vi "flip_tunnel.vi"() -> ()   [LabVIEW 2012]
uses:
  <vilib>/userdefined/High Color/IMAQdx.ctl
  <vilib>/vision/driver/IMAQdx.llb/IMAQdx Acquisition Mode.ctl
  <vilib>/Platform/TimedLoop/XDataNode/timing_clust.ctl
  <vilib>/Platform/TimedLoop/XDataNode/nitl_modes.ctl
  <vilib>/Platform/TimedLoop/XDataNode/wakeup.ctl
  <vilib>/vision/driver/IMAQdx.llb/IMAQdx Buffer Number Mode.ctl
  <vilib>/DAQmx/read.llb/DAQmx Read (Counter 1D DBL 1Chan NSamp).vi
  <vilib>/DAQmx/read.llb/DAQmx Read (Analog 1D Wfm NChan NSamp).vi
  <vilib>/DAQmx/create/channels.llb/DAQmx Create Channel (CI-Position-Angular Encoder).vi
  <vilib>/DAQmx/configure/timing.llb/DAQmx Timing (Sample Clock).vi
  <vilib>/DAQmx/create/channels.llb/DAQmx Create Channel (AI-Voltage-Basic).vi
  <vilib>/DAQmx/miscellaneous.llb/DAQmx Fill In Error Info.vi
  <vilib>/Utility/config.llb/Write Key (U32).vi
  <vilib>/Utility/config.llb/Write Key (Double).vi
  <vilib>/Utility/config.llb/Write Key (I32).vi
  <vilib>/Utility/config.llb/Write Key (String).vi
  <vilib>/platform/TimedLoop/XDataNode/XDataNode.xnode
  <resource>/objmgr/daqmx.rc
  <vilib>/vision/driver/NI_Vision_Acquisition_Software.lvlib
  <vilib>/Utility/config.llb/NI_LVConfig.lvlib
  <resource>/objmgr/imaqdx.rc
  <vilib>/Platform/TimedLoop/XDataNode/XDNodeRunTimeDep.lvlib
  <vilib>/vision/NI_Vision_Development_Module.lvlib
  <resource>/objmgr/IMAQImage.rc
panel:
  out "Speed (tunnel)":dbl(graph)
  out "Numeric":i32=1056
  out "Numeric 2":i32=1057
  out "Image CAM0- front view 3":T1(plugin-control)
  out "Lick":dbl[](graph)=[0.2311358645899357, 0.23014957542213182, 0.2311358645899357, 0.2308071015339834, 0.23047833847804877, 0.2308071015339834, 0.2311358645899357, 0.2311358645899357, 0.2308071015339834, 0.2308071015339834, 0.2308071015339834, 0.23047833847804877, 0.23014957542213182, 0.23047833847804877, 0.23047833847804877, 0.2308071015339834, 0.2308071015339834, 0.23014957542213182, 0.23047833847804877, 0.23047833847804877, 0.23047833847804877, 0.23014957542213182, 0.2298208123662325, 0.2298208123662325, 0.23047833847804877, 0.2298208123662325, 0.2298208123662325, 0.2298208123662325, 0.2298208123662325, 0.2291632862544866, 0.22949204931035078, 0.22949204931035078, 0.23014957542213182, 0.2298208123662325, 0.23014957542213182, 0.2298208123662325, 0.2298208123662325, 0.2298208123662325, 0.2298208123662325, 0.2298208123662325, 0.2298208123662325, 0.23014957542213182, 0.23014957542213182, 0.23014957542213182, 0.2298208123662325, 0.2298208123662325, 0.23047833847804877, 0.23047833847804877, 0.2298208123662325, 0.23047833847804877, 0.23014957542213182, 0.23014957542213182, 0.23014957542213182, 0.23014957542213182, 0.23014957542213182, 0.23047833847804877, 0.23014957542213182, 0.23047833847804877, 0.2308071015339834, 0.23047833847804877, 0.2298208123662325, 0.23047833847804877, 0.23047833847804877, 0.2308071015339834, 0.2308071015339834, 0.2308071015339834, 0.2311358645899357, 0.2311358645899357, 0.2311358645899357, 0.2308071015339834, 0.23047833847804877, 0.2311358645899357, 0.2311358645899357, 0.2308071015339834, 0.2308071015339834, 0.23179339070189353, 0.2308071015339834, 0.2311358645899357, 0.23146462764590575, 0.2311358645899357, 0.23146462764590575, 0.2311358645899357, 0.2311358645899357, 0.23146462764590575, 0.2311358645899357, 0.23146462764590575, 0.23146462764590575, 0.23146462764590575, 0.2311358645899357, 0.2311358645899357, 0.2311358645899357, 0.2311358645899357, 0.2311358645899357, 0.23146462764590575, 0.2308071015339834, 0.2308071015339834, 0.2308071015339834, 0.2308071015339834, 0.2308071015339834, 0.2311358645899357]
  in  "Optional Rectangle":i32[](array[numeric])=[200, 100, 550, 400]
  out "Image CAM0- front view 2":T1(plugin-control)
  out "Speed":dbl(graph)
  out "Image Type 2":i32(ring) items=["8 bits", "16 bits", "Float", "Complex", "RGB", "HSL"]
  out "Image Type":i32(ring) items=["8 bits", "16 bits", "Float", "Complex", "RGB", "HSL"]
  out "Image Size":cluster{"x":i32, "y":i32}={"x"=350, "y"=300}
  out "AISaveLoop 2":i32
  out "LEDDriver":dbl[](graph)=[-0.0036009546902470956, -0.0022859024861033913, -0.0016283763840546168, -0.0022859024861033913, -0.0026146655371335026, -0.0039297177412928146, -0.0039297177412928146, -0.00294342858816747, -0.00294342858816747, -0.0019571394350771064, -0.004587243843396215, -0.0052447699455157705, -0.00294342858816747, -0.0032721916392053243, -0.0039297177412928146, -0.0032721916392053243, -0.00294342858816747, -0.0022859024861033913, -0.0032721916392053243, -0.0032721916392053243, -0.0039297177412928146, -0.0039297177412928146, -0.00425848079234251, -0.0039297177412928146, -0.0036009546902470956, -0.0032721916392053243, -0.00425848079234251, -0.0039297177412928146, -0.0039297177412928146, -0.0039297177412928146, -0.0026146655371335026, -0.0036009546902470956, -0.0032721916392053243, -0.0026146655371335026, -0.0022859024861033913, -0.0032721916392053243, -0.0012996133330358927, -0.00294342858816747, -0.0022859024861033913, -0.0019571394350771064, -0.0019571394350771064, -0.00294342858816747, -0.0019571394350771064, -0.0016283763840546168, -0.0026146655371335026, -0.0032721916392053243, -0.0022859024861033913, -0.0032721916392053243, -0.0036009546902470956, -0.0019571394350771064, -0.0026146655371335026, -0.0039297177412928146, -0.00294342858816747, -0.00425848079234251, -0.0022859024861033913, -0.0022859024861033913, -0.0022859024861033913, -0.0026146655371335026, -0.0036009546902470956, -0.0026146655371335026, -0.0026146655371335026, -0.0026146655371335026, -0.0026146655371335026, -0.0026146655371335026, -0.00294342858816747, -0.0039297177412928146, -0.0039297177412928146, -0.00294342858816747, -0.00294342858816747, -0.00294342858816747, -0.0019571394350771064, -0.00294342858816747, -0.0019571394350771064, -0.0022859024861033913, -0.0019571394350771064, -0.0016283763840546168, -0.0036009546902470956, -0.0032721916392053243, -0.0022859024861033913, -0.0019571394350771064, -0.0009708502820209035, -0.0032721916392053243, -0.0026146655371335026, -0.00294342858816747, -0.0032721916392053243, -0.0022859024861033913, -0.0032721916392053243, -0.0026146655371335026, -0.0032721916392053243, -0.0022859024861033913, -0.0026146655371335026, -0.0026146655371335026, -0.0036009546902470956, -0.0039297177412928146, -0.0032721916392053243, -0.0026146655371335026, -0.0022859024861033913, -0.00294342858816747, -0.00294342858816747, -0.0032721916392053243]
  out "Position":dbl[](graph)=[-0.10288739642478602, -0.10288739642478602, -0.10288739642478602, -0.10288739642478602, -0.10255863337117274, -0.10255863337117274, -0.10255863337117274, -0.10288739642478602, -0.10255863337117274, -0.10288739642478602, -0.10288739642478602, -0.10321615947841241, -0.10288739642478602, -0.10288739642478602, -0.10354492253205194, -0.10321615947841241, -0.10255863337117274, -0.10321615947841241, -0.10321615947841241, -0.10354492253205194, -0.10321615947841241, -0.10387368558570464, -0.10354492253205194, -0.10387368558570464, -0.10354492253205194, -0.10321615947841241, -0.10321615947841241, -0.10354492253205194, -0.10354492253205194, -0.10354492253205194, -0.10288739642478602, -0.10420244863937056, -0.10354492253205194, -0.10321615947841241, -0.10387368558570464, -0.10321615947841241, -0.10354492253205194, -0.10354492253205194, -0.10321615947841241, -0.10321615947841241, -0.10321615947841241, -0.10321615947841241, -0.10321615947841241, -0.10288739642478602, -0.10321615947841241, -0.10387368558570464, -0.10321615947841241, -0.10321615947841241, -0.10321615947841241, -0.10321615947841241, -0.10288739642478602, -0.10321615947841241, -0.10387368558570464, -0.10321615947841241, -0.10354492253205194, -0.10354492253205194, -0.10354492253205194, -0.10354492253205194, -0.10354492253205194, -0.10321615947841241, -0.10288739642478602, -0.10321615947841241, -0.10321615947841241, -0.10288739642478602, -0.10288739642478602, -0.10255863337117274, -0.10321615947841241, -0.10288739642478602, -0.10321615947841241, -0.10321615947841241, -0.10288739642478602, -0.10255863337117274, -0.10255863337117274, -0.10288739642478602, -0.10288739642478602, -0.10354492253205194, -0.10288739642478602, -0.10321615947841241, -0.10288739642478602, -0.10288739642478602, -0.10255863337117274, -0.10255863337117274, -0.10255863337117274, -0.10255863337117274, -0.10255863337117274, -0.10288739642478602, -0.10222987031757254, -0.10222987031757254, -0.10255863337117274, -0.10288739642478602, -0.10288739642478602, -0.10255863337117274, -0.10255863337117274, -0.10255863337117274, -0.10255863337117274, -0.10255863337117274, -0.10288739642478602, -0.10288739642478602, -0.10288739642478602, -0.10288739642478602]
  out "Punish":dbl[](graph)=[-0.13181854519755057, -0.13181854519755057, -0.13214730825244975, -0.1314897821426672, -0.13214730825244975, -0.13214730825244975, -0.13247607130736472, -0.13181854519755057, -0.13247607130736472, -0.13214730825244975, -0.13181854519755057, -0.13214730825244975, -0.13214730825244975, -0.13247607130736472, -0.13214730825244975, -0.13214730825244975, -0.13247607130736472, -0.13280483436229554, -0.13280483436229554, -0.13247607130736472, -0.13247607130736472, -0.13214730825244975, -0.13247607130736472, -0.13247607130736472, -0.13247607130736472, -0.13280483436229554, -0.13247607130736472, -0.13247607130736472, -0.13280483436229554, -0.13280483436229554, -0.13247607130736472, -0.13247607130736472, -0.13247607130736472, -0.13247607130736472, -0.13313359741724223, -0.13214730825244975, -0.13247607130736472, -0.13247607130736472, -0.13247607130736472, -0.13280483436229554, -0.13280483436229554, -0.13247607130736472, -0.13280483436229554, -0.13214730825244975, -0.13280483436229554, -0.13247607130736472, -0.13247607130736472, -0.13247607130736472, -0.13280483436229554, -0.13247607130736472, -0.13247607130736472, -0.13214730825244975, -0.13247607130736472, -0.13280483436229554, -0.13247607130736472, -0.13247607130736472, -0.13247607130736472, -0.13181854519755057, -0.13247607130736472, -0.13214730825244975, -0.13247607130736472, -0.13214730825244975, -0.13247607130736472, -0.13181854519755057, -0.13247607130736472, -0.13214730825244975, -0.13214730825244975, -0.13181854519755057, -0.13214730825244975, -0.13214730825244975, -0.13214730825244975, -0.13181854519755057, -0.13181854519755057, -0.13214730825244975, -0.13181854519755057, -0.13214730825244975, -0.1311610190877996, -0.1314897821426672, -0.1314897821426672, -0.13181854519755057, -0.1314897821426672, -0.13181854519755057, -0.13214730825244975, -0.1314897821426672, -0.1314897821426672, -0.1314897821426672, -0.13214730825244975, -0.13181854519755057, -0.13214730825244975, -0.13181854519755057, -0.13214730825244975, -0.13181854519755057, -0.13214730825244975, -0.13181854519755057, -0.13247607130736472, -0.1314897821426672, -0.13214730825244975, -0.13181854519755057, -0.13181854519755057, -0.13181854519755057]
  out "FramePulse":dbl[](graph)=[-0.0019571394350771064, -0.0016283763840546168, -0.0006420872310096188, -0.0012996133330358927, -0.0006420872310096188, -0.0012996133330358927, -0.0022859024861033913, -0.0022859024861033913, -0.0022859024861033913, -0.0026146655371335026, -0.00425848079234251, -0.0032721916392053243, -0.0019571394350771064, -0.0039297177412928146, -0.00425848079234251, -0.0006420872310096188, -0.0016283763840546168, -0.0019571394350771064, -0.0036009546902470956, -0.0022859024861033913, -0.0036009546902470956, -0.0022859024861033913, -0.0032721916392053243, -0.0022859024861033913, -0.0032721916392053243, -0.00294342858816747, -0.0036009546902470956, -0.0022859024861033913, -0.0016283763840546168, -0.0026146655371335026, -0.0016283763840546168, -0.0026146655371335026, -0.00294342858816747, -0.0006420872310096188, -0.0019571394350771064, -0.00294342858816747, -0.0009708502820209035, -0.0022859024861033913, -0.0009708502820209035, -0.0019571394350771064, -0.0012996133330358927, -0.0039297177412928146, -0.0026146655371335026, -0.0012996133330358927, -0.0012996133330358927, -0.0019571394350771064, -0.00294342858816747, -0.0022859024861033913, -0.00294342858816747, -0.0026146655371335026, -0.0019571394350771064, -0.0019571394350771064, -0.00294342858816747, -0.0036009546902470956, -0.0012996133330358927, -0.00031332418000200855, -0.0016283763840546168, -0.0019571394350771064, -0.00294342858816747, -0.0026146655371335026, -0.0036009546902470956, -0.0022859024861033913, -0.0019571394350771064, -0.0006420872310096188, -0.0009708502820209035, -0.0026146655371335026, -0.0036009546902470956, -0.0009708502820209035, -0.0026146655371335026, -0.0032721916392053243, -0.0019571394350771064, -0.00294342858816747, -0.0019571394350771064, -0.0022859024861033913, -0.00294342858816747, -0.0022859024861033913, -0.0036009546902470956, -0.0016283763840546168, -0.0026146655371335026, -0.0016283763840546168, -0.0019571394350771064, -0.0022859024861033913, -0.0019571394350771064, -0.0016283763840546168, -0.0022859024861033913, -0.0012996133330358927, -0.0012996133330358927, -0.0016283763840546168, -0.0012996133330358927, -0.0022859024861033913, -0.0026146655371335026, -0.0016283763840546168, -0.0032721916392053243, -0.0036009546902470956, -0.0019571394350771064, -0.0012996133330358927, -0.0016283763840546168, -0.0012996133330358927, -0.0019571394350771064, -0.0019571394350771064]
  out "Stim ID":dbl[](graph)=[-0.2067765221829541, -0.2067765221829541, -0.2067765221829541, -0.2067765221829541, -0.2064477591236867, -0.20710528524224417, -0.2067765221829541, -0.2067765221829541, -0.20710528524224417, -0.20710528524224417, -0.20710528524224417, -0.2067765221829541, -0.2067765221829541, -0.20710528524224417, -0.2067765221829541, -0.20710528524224417, -0.20710528524224417, -0.20710528524224417, -0.20743404830155698, -0.2067765221829541, -0.20710528524224417, -0.20710528524224417, -0.20710528524224417, -0.2067765221829541, -0.20743404830155698, -0.2067765221829541, -0.20710528524224417, -0.2064477591236867, -0.20710528524224417, -0.2067765221829541, -0.2067765221829541, -0.20710528524224417, -0.2067765221829541, -0.2064477591236867, -0.2067765221829541, -0.20710528524224417, -0.20710528524224417, -0.20743404830155698, -0.20710528524224417, -0.2067765221829541, -0.2067765221829541, -0.20710528524224417, -0.2067765221829541, -0.2067765221829541, -0.2067765221829541, -0.20710528524224417, -0.2067765221829541, -0.2067765221829541, -0.2064477591236867, -0.20743404830155698, -0.2067765221829541, -0.20710528524224417, -0.2067765221829541, -0.2067765221829541, -0.20710528524224417, -0.20710528524224417, -0.20743404830155698, -0.20743404830155698, -0.20710528524224417, -0.20710528524224417, -0.2067765221829541, -0.20710528524224417, -0.20710528524224417, -0.2067765221829541, -0.2064477591236867, -0.20710528524224417, -0.2067765221829541, -0.20743404830155698, -0.2067765221829541, -0.2064477591236867, -0.2064477591236867, -0.2067765221829541, -0.2064477591236867, -0.2067765221829541, -0.20710528524224417, -0.2064477591236867, -0.20710528524224417, -0.2067765221829541, -0.2067765221829541, -0.2067765221829541, -0.2067765221829541, -0.2067765221829541, -0.20710528524224417, -0.2067765221829541, -0.2067765221829541, -0.2067765221829541, -0.2067765221829541, -0.2067765221829541, -0.2064477591236867, -0.2067765221829541, -0.20743404830155698, -0.2064477591236867, -0.2067765221829541, -0.2064477591236867, -0.20743404830155698, -0.20710528524224417, -0.20710528524224417, -0.2064477591236867, -0.20743404830155698, -0.2067765221829541]
  out "Photodiode":dbl[](graph)=[1.0477834277971203, 1.0444957958656487, 1.0550162180791747, 1.0579750868439877, 1.0694817987797698, 1.0790159316147676, 1.088878827735934, 1.0796734580201486, 1.0970979079034913, 1.099728013569978, 1.098741723944312, 1.0842761428685865, 1.0895363541471035, 1.0800022212229832, 1.0497560069604706, 1.0283863995350169, 1.048769717378376, 1.0435095062880182, 1.0481121909907791, 1.0494272437663457, 1.0329890841783826, 1.0517285861271792, 1.0395643479858325, 1.0602764292218856, 1.0369342424584334, 1.0803309844259137, 1.0803309844259137, 1.0892075909414702, 1.088878827735934, 1.099728013569978, 1.0957828550725925, 1.0895363541471035, 1.0763858259970813, 1.0760570627953017, 1.073426957184508, 1.0550162180791747, 1.0339753737471549, 1.0435095062880182, 1.0408794007517477, 1.0438382694804689, 1.0227974253492698, 1.0467971382167025, 1.0553449812748896, 1.0648791139915486, 1.0494272437663457, 1.0760570627953017, 1.0878925381199063, 1.0908514069706063, 1.0898651173528338, 1.0517285861271792, 1.0924952230021696, 1.0901938805586608, 1.0829610900528213, 1.064550350793101, 1.0599476660247606, 1.0586326132372021, 1.0553449812748896, 1.0402218743686054, 1.0339753737471549, 1.0405506375601303, 1.0438382694804689, 1.038578058412366, 1.0513998229324943, 1.0513998229324943, 1.0655366403887276, 1.0711256147800765, 1.0790159316147676, 1.0875637749147575, 1.0763858259970813, 1.100056776778729, 1.0872350117097054, 1.0859199588904642, 1.0842761428685865, 1.0744132467878387, 1.052714875711795, 1.0507422965434046, 1.0507422965434046, 1.045810848637122, 1.0303589786656915, 1.0362767160775053, 1.0379205320305165, 1.0264138204076296, 1.0441670326730124, 1.0612627188138266, 1.064221587594748, 1.0727694307827649, 1.0704680883796682, 1.0892075909414702, 1.0892075909414702, 1.081974800442009, 1.073426957184508, 1.0892075909414702, 1.081974800442009, 1.0707968515798247, 1.0237837149095494, 1.0467971382167025, 1.0513998229324943, 1.0313452682322635, 1.03759176883973, 1.0178659775601138]
  out "Elapsed time":u32=37 format="%<%H:%M:%S>t"
  in  "?":enum32{"CodePerformance", "SetPath"}(tab)=enum."SetPath"
  out "CamerasOK? TaskEnd OK?":errorcluster
  in  "SetPath OK?":errorcluster
  out "AcqLoopRes[ms]":u32=100
  out "SaveLoopRes[ms]":u32=100
  out "AISaveLoop":i32=373
  out "AIAcqLoop":i32=372
  out "Cam2AcqRes[ms]":u32=40
  out "# elements in queue":i32
  out "Cam1AcqRes[ms]":u32=63
  out "error out":errorcluster
  out "Buffer Number  2":u32=1189
  out "Frame Rate 2":dbl=28.403525954946133
  out "Buffer Number":u32=47166
  out "Frame Rate":dbl=15.968063872255488
  in  "File prefix":string="T7"
  in  "Path":path=path "D:/Kelly_Raja"
  out "FileName":string="20170427_193446_T7"
  out "byte order (0:big-endian, network order)":T2(ring)
  out "NumChans":u32=12
  in  "SaveData":bool
  in  "all stop":bool=TRUE
  in  "start":bool=TRUE
  in  "samples per channel":i32=100
  in  "rate":dbl=1000.0 format="%0.2f"
  out "Acquired Frames CAM0":dbl=28.431372549019606
  out "SaveLoopRes[ms] 2":u32=348059
  out "# elements in queue 2":i32
  out "Number of trials":dbl
  out "?":T1(plugin-control)
  out "?":T1(plugin-control)
  out "Reward":dbl[](graph)=[1.543887100195785e-05, -0.00031332418000200855, 1.543887100195785e-05, 1.543887100195785e-05, -0.00031332418000200855, -0.00031332418000200855, 0.0003442019220023107, 1.543887100195785e-05, 0.0003442019220023107, 0.0003442019220023107, 1.543887100195785e-05, 0.0003442019220023107, 1.543887100195785e-05, 1.543887100195785e-05, 1.543887100195785e-05, -0.00031332418000200855, -0.00031332418000200855, 1.543887100195785e-05, -0.00031332418000200855, 0.0003442019220023107, -0.0006420872310096188, 1.543887100195785e-05, 1.543887100195785e-05, 0.0003442019220023107, 1.543887100195785e-05, 0.0003442019220023107, 0.0003442019220023107, -0.0006420872310096188, 1.543887100195785e-05, 1.543887100195785e-05, 0.0003442019220023107, -0.00031332418000200855, 1.543887100195785e-05, 1.543887100195785e-05, 1.543887100195785e-05, 1.543887100195785e-05, 0.0003442019220023107, 1.543887100195785e-05, 1.543887100195785e-05, 0.0003442019220023107, -0.00031332418000200855, 1.543887100195785e-05, 1.543887100195785e-05, 1.543887100195785e-05, 1.543887100195785e-05, 0.0003442019220023107, -0.00031332418000200855, -0.0006420872310096188, 1.543887100195785e-05, 1.543887100195785e-05, 1.543887100195785e-05, 1.543887100195785e-05, 1.543887100195785e-05, 0.0003442019220023107, 1.543887100195785e-05, 1.543887100195785e-05, -0.00031332418000200855, -0.00031332418000200855, 1.543887100195785e-05, -0.00031332418000200855, -0.00031332418000200855, 1.543887100195785e-05, 1.543887100195785e-05, 1.543887100195785e-05, 1.543887100195785e-05, 0.0003442019220023107, 1.543887100195785e-05, -0.00031332418000200855, -0.00031332418000200855, -0.00031332418000200855, 1.543887100195785e-05, 0.0003442019220023107, 1.543887100195785e-05, -0.00031332418000200855, 1.543887100195785e-05, 1.543887100195785e-05, 0.0006729649729990802, 1.543887100195785e-05, 1.543887100195785e-05, 0.0003442019220023107, -0.00031332418000200855, -0.00031332418000200855, 1.543887100195785e-05, 0.0003442019220023107, 1.543887100195785e-05, 1.543887100195785e-05, -0.00031332418000200855, 1.543887100195785e-05, 1.543887100195785e-05, -0.00031332418000200855, 0.0003442019220023107, -0.00031332418000200855, 1.543887100195785e-05, 1.543887100195785e-05, 1.543887100195785e-05, 1.543887100195785e-05, 1.543887100195785e-05, -0.00031332418000200855, -0.00031332418000200855, -0.00031332418000200855]
  out "dup path":path=path "D:/Kelly_Raja"
  out "created path":path=path "D:/Kelly_Raja"
  # "RecordAI_VI (orsolici, 2016)"
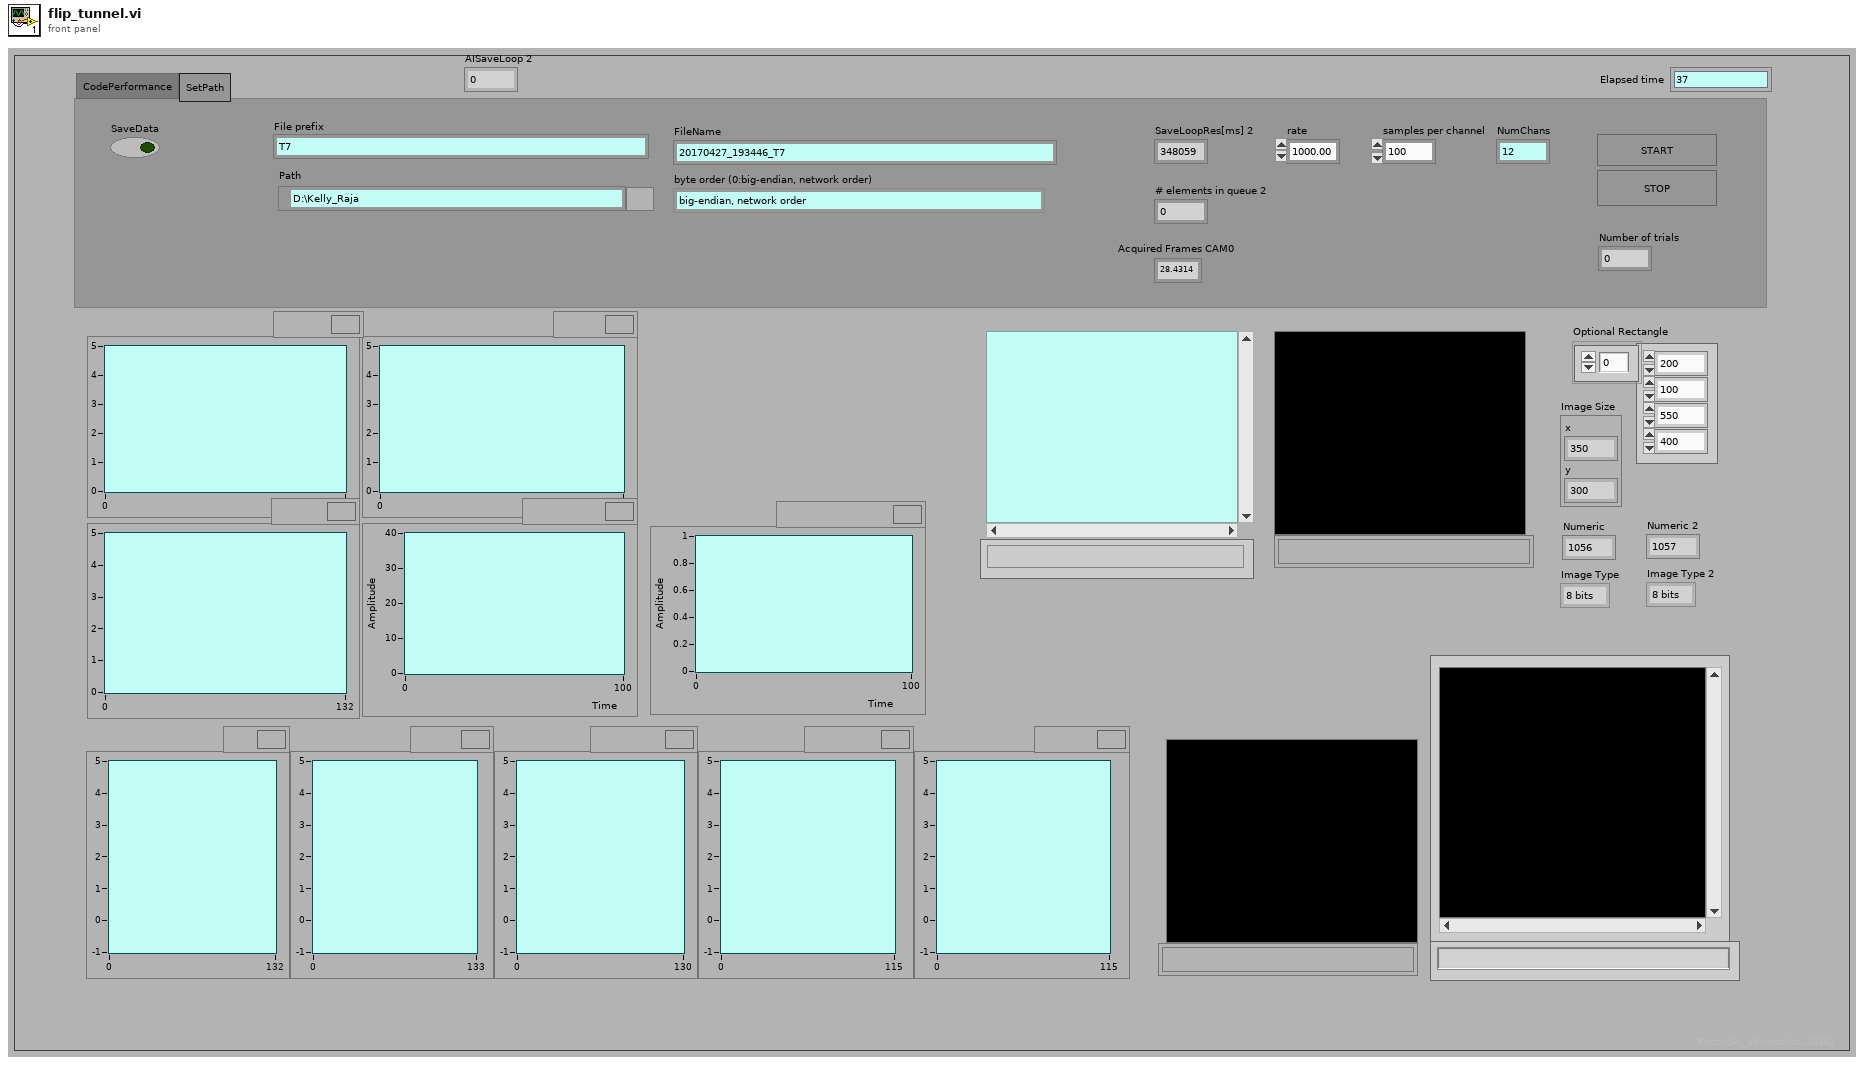
[diagram p1: front panel]
types:
  T1 = typedef "IMAQ Image.ctl" = refnum<image>
  T2 = enum16{"big-endian, network order", "native, host order", "little-endian"}
  T3 = typedef "IMAQdx.ctl" = refnum<k21>
  T4 = typedef "Image Type" = u32
  T5 = cluster{i32, "millisecond timer value":u32, "Buffer Number Out":u32, "Image Pixels (U8)":u8[][]}
  T6 = cluster{"data":waveform(dbl)[], "data":dbl[], "millisecond timer value":u32, i32}
  T7 = typedef "NI_Vision_Acquisition_Software.lvlib/IMAQdx Acquisition Mode.ctl" = enum32{"One Shot", "Continuous"}
  T8 = cluster{"New Image":T1, "Session Out":T3, "error out":errorcluster}
  T9 = cluster{"task out":refnum<k21>, "error out":errorcluster, "task out":refnum<k21>, "error out":errorcluster}
  T10 = cluster{"Session Out":T3, "New Image":T1, "New Image":T1, "error out":errorcluster}
  T11 = typedef "XDNodeRunTimeDep.lvlib/timing_clust.ctl" = cluster{"Expected End [f-1]":u64, "Actual End [f-1]":u64, "Finished Late? [f-1]":bool, "Expected End [i-1]":u64, "Actual End [i-1]":u64, "Finished Late? [i-1]":bool, "Expected Start [i]":u64, "Actual Start [i]":u64, "Expected Start [f]":u64, "Actual Start [f]":u64, "Source Name":string, "Structure Name":string, "Period":i64, "Deadline":i64, "Offset":i64, "Start":i64, "Priority":i32, "Timeout":i32, "Mode":T12, "Wakeup Reason":T13, "Error":errorcluster, "Source Type":string, "Secondary Source Type":string, "Global End Time":u64, "Global Start Time":u64, "Frame Duration":u64, "Iteration Duration":u64, "Assigned CPU":i32, "I/O Scan Engine Mode":u32}
  T12 = typedef "XDNodeRunTimeDep.lvlib/nitl_modes.ctl" = enum32{"No Change", "Process missed periods, maintain original phase", "Discard missed periods, maintain original phase", "Process missed periods, ignore original phase", "Discard missed periods, ignore original phase"}
  T13 = typedef "XDNodeRunTimeDep.lvlib/wakeup.ctl" = enum32{"Normal", "Aborted", "Asynchronous wakeup", "Timing source error", "Timed loop error", "Timeout"}
  T14 = enum16{"open", "replace", "create", "open or create", "replace or create", "replace or create with confirmation"}
  T15 = cluster{refnum<file>[], "refnum out":refnum<file>, "refnum out":refnum<file>, "refnum out":refnum<file>}
  T16 = typedef "NI_Vision_Acquisition_Software.lvlib/IMAQdx Buffer Number Mode.ctl" = enum32{"Next", "Last", "Buffer Number"}
  T17 = cluster{"Image Out":T1, "Session Out":T3, "error out":errorcluster}
  T18 = cluster{"Session Out":T3, "error out":errorcluster, "New Image":T1}
  T19 = cluster{cluster{"Image Out":T1, "Session Out":T3, "error out":errorcluster}, cluster{"Image Out":T1, "Session Out":T3, "error out":errorcluster}}
  T20 = typedef "NI_LVConfig.lvlib/Config Data RefNum.ctl" = refnum<k1>
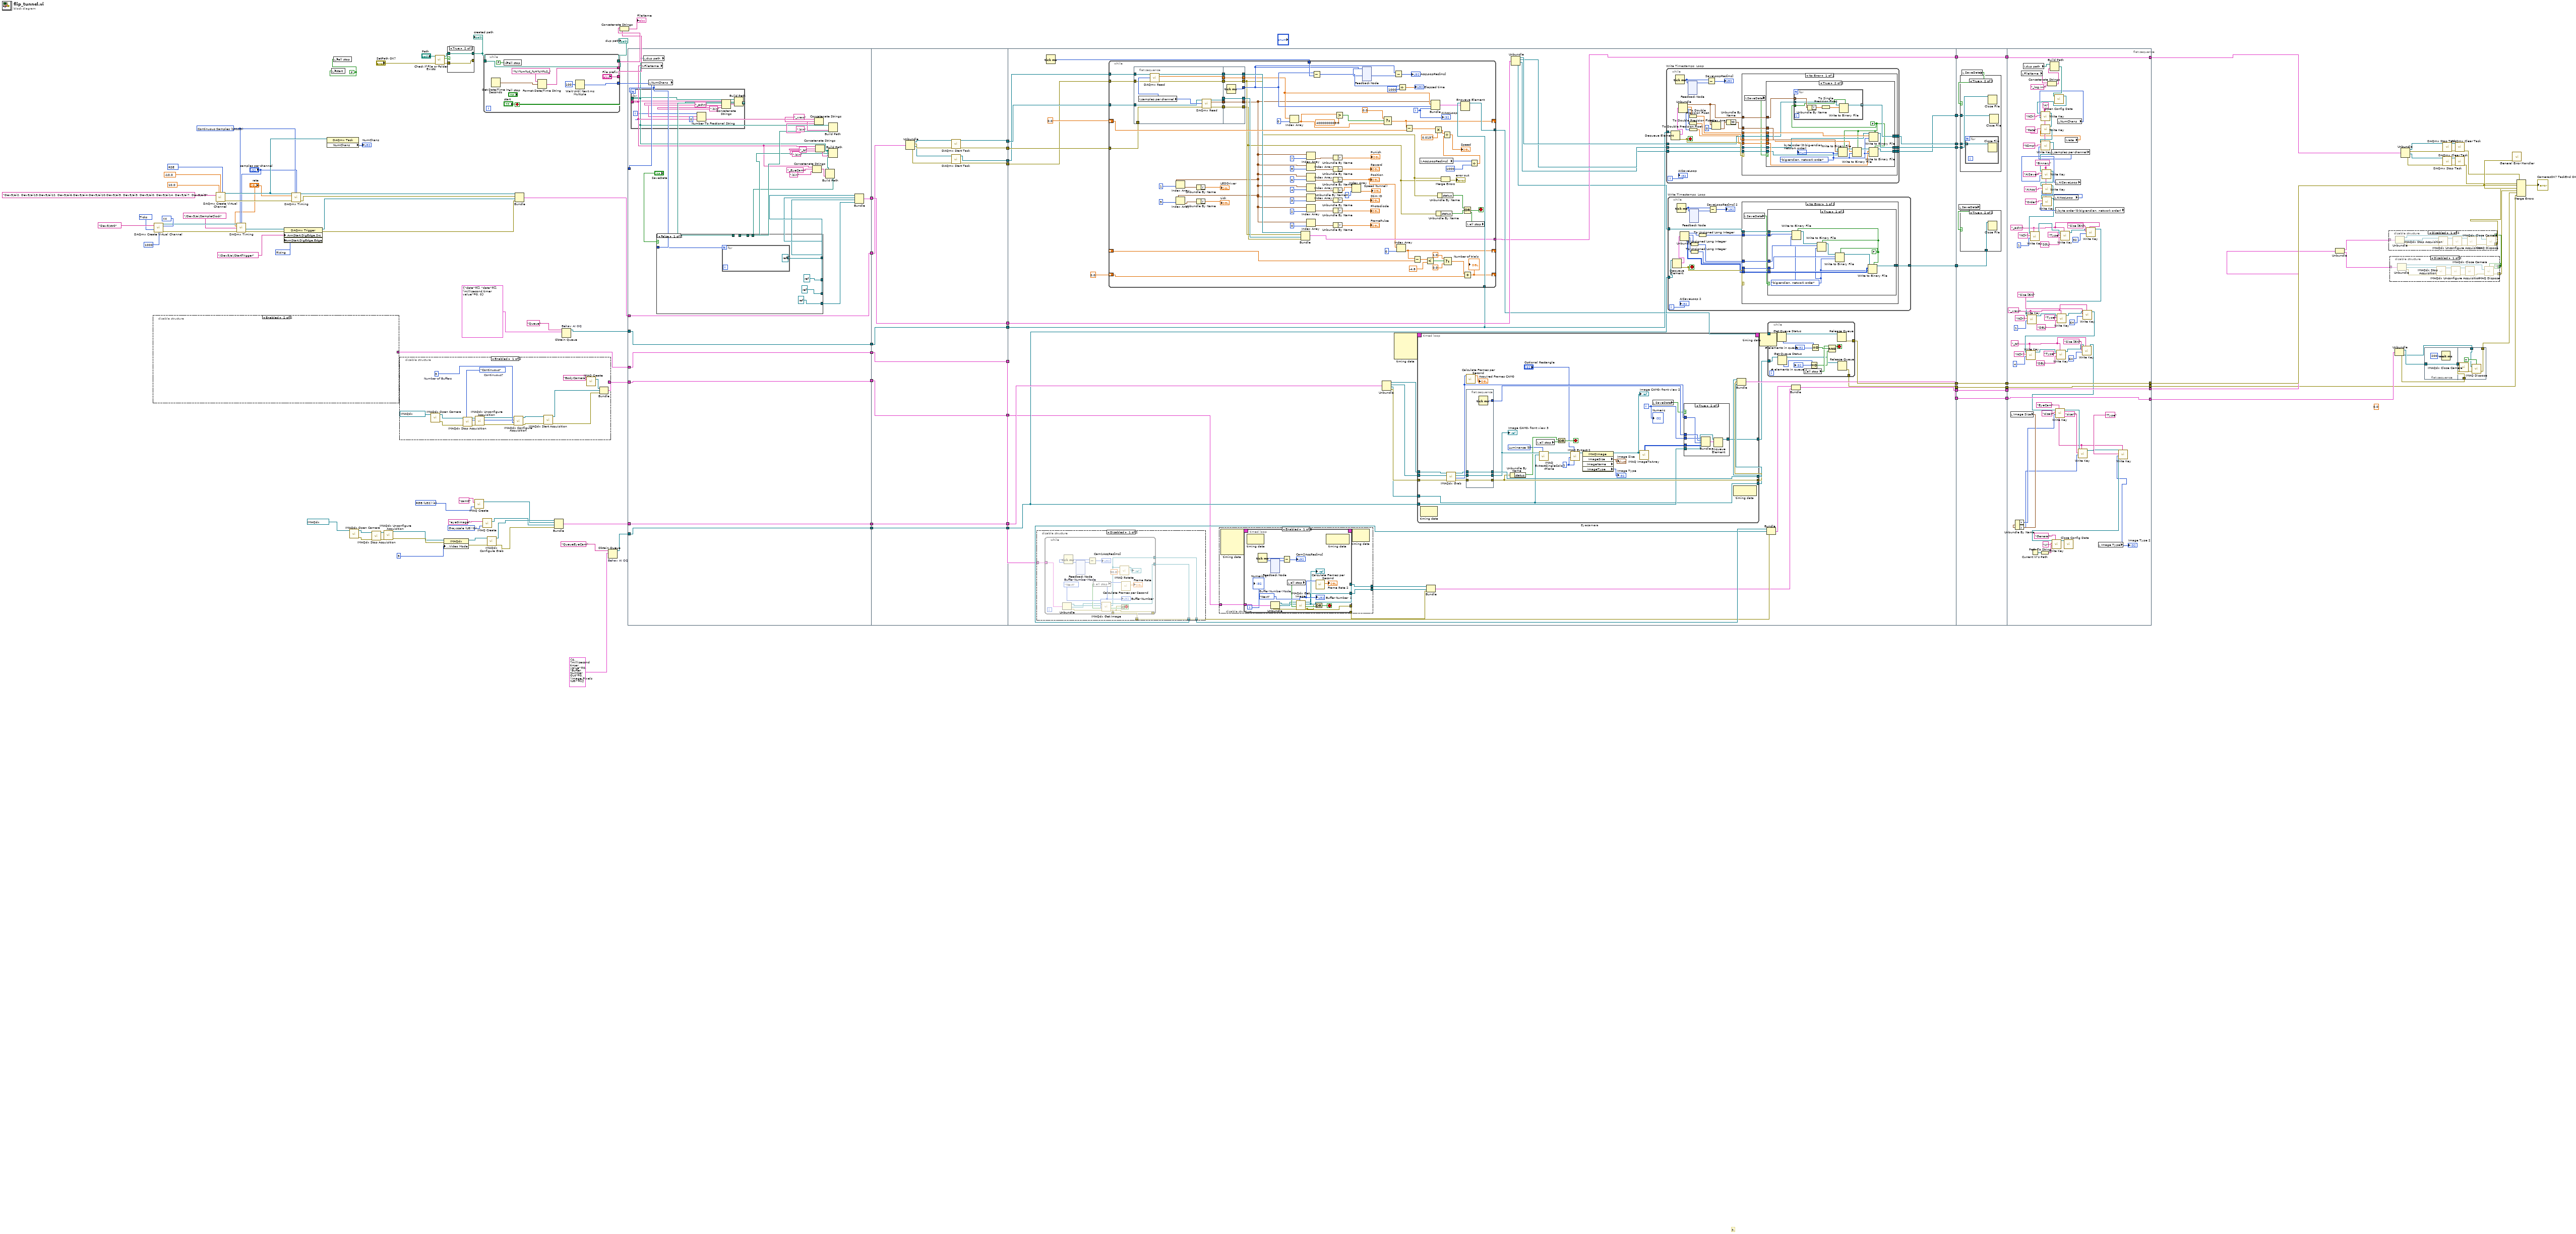
[diagram p0: block diagram]
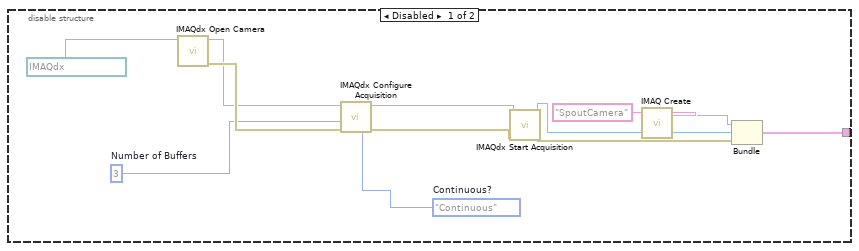
[diagram p5: hidden frame]
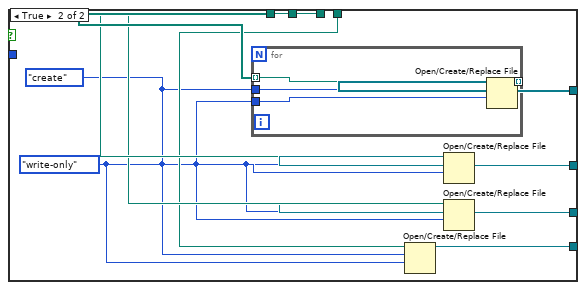
[diagram p6: hidden frame]
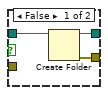
[diagram p16: hidden frame]
diagram:
  w30 = T4 0 items=["Grayscale (U8)", "Grayscale (I16)", "Grayscale (SGL)", "Complex (CSG)", "RGB (U32)", "HSL (U32)", "RGB (U64)", "Grayscale (U16)"] ("Image Type")
  w32 = T4 4 items=["Grayscale (U8)", "Grayscale (I16)", "Grayscale (SGL)", "Complex (CSG)", "RGB (U32)", "HSL (U32)", "RGB (U64)", "Grayscale (U16)"] ("Image Type")
  (unwired) 0.0 ("data")
  w59 = 10304 items=["Degrees"=10146, "Radians"=10273, "Ticks"=10304, "From Custom Scale"=10065] ("units")
  w2 = 10123 items=["Finite Samples"=10178, "Continuous Samples"=10123, "Hardware Timed Single Point"=12522] ("sample mode")
  w73 = 10083 items=["default"=-1, "RSE"=10083, "NRSE"=10078, "Differential"=10106, "Pseudodifferential"=12529] ("input terminal configuration")
  w70 = 10092 items=["X1"=10090, "X2"=10091, "X4"=10092, "Two Pulse Counting"=10313] ("E1 decoding type")
  w63 = 10280 items=["Rising"=10280, "Falling"=10171] ("ArmStart.DigEdge.Edge")
  w13 = FALSE
  # "3."
  n1 = disable-structure shown="Enabled" {
    disable-tunnel: [w130 _] -> w100
    frame Disabled {
      w123 = IMAQdx_Acquisition_Mode."Continuous"  # Continuous?
      w133 = u32 3  # Number of Buffers
      n2 = call <vilib>:"IMAQdx Open Camera.vi"("Session In"=T3 "spout camera" ("Camera1")) -> ("error out"=w134:errorcluster, "Session Out"=w129:T3)  [unwired: 2 in, 7 out]
      n3 = call <vilib>:"IMAQdx Configure Acquisition.vi"("error in"=w134, "Number of Buffers"=w133, "Continuous?"=w123, "Session In"=w129) -> ("error out"=w124:errorcluster, "Session Out"=w127:T3)  [unwired: 6 out]
      n4 = call <vilib>:"IMAQdx Start Acquisition.vi"("error in"=w124, "Session In"=w127) -> ("error out"=w125:errorcluster, "Session Out"=w126:T3)  [unwired: 8 out]
      n5 = call "IMAQ Create"("Image Name"="SpoutCamera") -> ("New Image"=w131:T1)  [unwired: 3 in, 2 out]
      n6 = Bundle("New Image"=w131, "Session Out"=w126, "error out"=w125) -> (w130:T8)  [unwired: 1 in]
    }
    frame Enabled {
    }
  }
  n7 = call-poly <vilib>:"DAQmx Create Virtual Channel.vi"("counter"=tag "Dev5/ctr0" ("E1 counter"), "decoding type"=w70, "units"=w59, "pulses per revolution"=u32 1000 ("E1 pulses per revolution")) -> ("task out"=w68:refnum<k21>, "error out"=w67:errorcluster)  [unwired: 10 in]
  n8 = call-poly <vilib>:"DAQmx Create Virtual Channel.vi"("maximum value"=10.0, "minimum value"=-10.0, "input terminal configuration"=w73, "physical channels"=tag "Dev5/ai2, Dev5/ai13,Dev5/ai12, Dev5/ai6,Dev5/ai4,Dev5/ai10,Dev5/ai5, Dev5/ai3, Dev5/ai0, Dev5/ai14, Dev5/ai7, Dev5/ai9" ("Analogue Input Channel")) -> ("task out"=w62:refnum<k21>, "error out"=w72:errorcluster)  [unwired: 10 in]
  n9 = call-poly <vilib>:"DAQmx Timing.vi"("task/channels in"=w68, "sample mode"=w2, "samples per channel"="samples per channel", "rate"="rate", "source"=tag "/Dev5/ai/SampleClock", "error in"=w67) -> ("task out"=w65:refnum<k21>, "error out"=w64:errorcluster)  [unwired: 8 in]
  n10 = property class="DAQmx Trigger"(reference=w65, error in=w64, "ArmStart.DigEdge.Src"=tag "/Dev5/ai/StartTrigger", "ArmStart.DigEdge.Edge"=w63) -> (reference out=w56:refnum<k21>, error out=w55:errorcluster)
  n11 = call-poly <vilib>:"DAQmx Timing.vi"("task/channels in"=w62, "sample mode"=w2, "samples per channel"="samples per channel", "rate"="rate", "error in"=w72) -> ("task out"=w58:refnum<k21>, "error out"=w57:errorcluster)  [unwired: 9 in]
  n12 = property class="DAQmx Task"(reference=w62) -> ("NumChans"=→"NumChans":u32)  [unwired: 1 in, 2 out]
  n13 = local write "start"(w13) -> ()
  n14 = local write "all stop"(w13) -> ()
  n15 = call <vilib>:"IMAQdx Open Camera.vi"("Session In"=T3 "eyecam2") -> ("error out"=w5:errorcluster, "Session Out"=w7:T3)  [unwired: 2 in, 7 out]
  n16 = call <vilib>:"IMAQdx Stop Acquisition.vi"("error in"=w5, "Session In"=w7) -> ("error out"=w4:errorcluster, "Session Out"=w6:T3)  [unwired: 8 in]
  n17 = call <vilib>:"IMAQdx Unconfigure Acquisition.vi"("error in"=w4, "Session In"=w6) -> ("error out"=w34:errorcluster, "Session Out"=w33:T3)  [unwired: 8 out]
  n18 = disable-structure shown="Enabled" {
    disable-tunnel: [w141 _] -> w10
    frame Enabled {
      w143 = u32 3  # Number of Buffers
      w145 = IMAQdx_Acquisition_Mode."Continuous"  # Continuous?
      n19 = call <vilib>:"IMAQdx Open Camera.vi"("Session In"=T3 "mousecam" ("Camera2")) -> ("error out"=w137:errorcluster, "Session Out"=w138:T3)  [unwired: 2 in, 7 out]
      n20 = call <vilib>:"IMAQdx Stop Acquisition.vi"("error in"=w137, "Session In"=w138) -> ("error out"=w140:errorcluster, "Session Out"=w139:T3)  [unwired: 8 in]
      n21 = call <vilib>:"IMAQdx Unconfigure Acquisition.vi"("error in"=w140, "Session In"=w139) -> ("error out"=w135:errorcluster, "Session Out"=w136:T3)  [unwired: 8 out]
      n22 = call <vilib>:"IMAQdx Configure Acquisition.vi"("error in"=w135, "Number of Buffers"=w143, "Continuous?"=w145, "Session In"=w136) -> ("error out"=w148:errorcluster, "Session Out"=w147:T3)  [unwired: 6 out]
      n23 = call <vilib>:"IMAQdx Start Acquisition.vi"("error in"=w148, "Session In"=w147) -> ("error out"=w149:errorcluster, "Session Out"=w150:T3)  [unwired: 8 out]
      n24 = call "IMAQ Create"("Image Name"="BodyCamera") -> ("New Image"=w144:T1)  [unwired: 3 in, 2 out]
      n25 = Bundle("New Image"=w144, "Session Out"=w150, "error out"=w149) -> (w141:T8)  [unwired: 1 in]
    }
    frame Disabled {
    }
  }
  n26 = call <vilib>:"Check if File or Folder Exists.vi"("error in (no error)"="SetPath OK?", "path"="Path") -> ("error out"=w118:errorcluster, "file or folder exists?"=w122:bool, "dup path"=w121:path)  [unwired: 7 in]
  n27 = property class="IMAQdx"(reference=w33, error in=w34, "Acquisition Attributes:Video Mode"=u32 5 ("VideoMode")) -> (reference out=w36:T3, error out=w35:errorcluster)
  n28 = case shown="True" w122 {
    tunnel: w121 -> [w153 w155]
    tunnel: [w152 w155] -> w119
    tunnel: w118 -> [_ w154]
    tunnel: [w151 w154] -> _
    frame False {
      n29 = Create Folder(path (use dialog)=w153) -> (created path=w152:path, error out=w151:errorcluster)  [unwired: 2 in, 1 out]
    }
    frame True {
    }
  }
  "created path" <- w119
  n30 = call "IMAQ Create"("Image Name"="cam0", "Image Type"=w32) -> ("New Image"=w41:T1)  [unwired: 2 in, 2 out]
  n31 = call "IMAQ Create"("Image Name"="eye0image", "Image Type"=w30) -> ("New Image"=w40:T1)  [unwired: 3 in, 1 out]
  n32 = while {
    tunnel: w119 -> [w156]
    tunnel: [w159] -> w102
    tunnel: ["File prefix"] -> w116
    tunnel: [w161] -> w117
    tunnel: [w156] -> w114
    stop <- "start" stop-if-true
    n33 = Get Date/Time In Seconds() -> (seconds since 1Jan1904=w157:timestamp)
    n34 = local write "all stop"(FALSE ("stop")) -> ()
    n35 = Format Date/Time String(time format string (%c)="%Y%m%d_%H%M%S_", seconds (now)=w157) -> (date/time string=w161:string)  [unwired: 1 in]
    n36 = Wait Until Next ms Multiple(millisecond multiple=u32 100) -> (millisecond timer value=w159:u32)
  }
  "dup path" <- w114
  n37 = call <vilib>:"IMAQdx Configure Grab.vi"("error in"=w35, "Session In"=w36) -> ("error out"=w53:errorcluster, "Session Out"=w42:T3)  [unwired: 1 in, 7 out]
  n38 = Bundle("task out"=w58, "error out"=w57, "task out"=w56, "error out"=w55) -> (w61:T9)  [unwired: 1 in]
  n39 = Bundle("Session Out"=w42, "New Image"=w41, "New Image"=w40, "error out"=w53) -> (w52:T10)  [unwired: 1 in]
  n40 = Obtain Queue "Behav AI OQ"(name (unnamed)="Queue", element data type=T6 {"data"=[], "data"=[], "millisecond timer value"=0, 0} ("cluster")) -> (queue out=w110:refnum<queue>)  [unwired: 3 in, 2 out]
  n41 = Obtain Queue "Behav AI OQ"(name (unnamed)="QueueEyeCam", element data type=T5 {0, "millisecond timer value"=0, "Buffer Number Out"=0, "Image Pixels (U8)"=[]} ("output cluster")) -> (queue out=w45:refnum<queue>)  [unwired: 3 in, 2 out]
  n42 = Concatenate Strings(w117, w116) -> (→"FileName":string)
  n43 = flat-sequence {
    tunnel: [w186] -> w111
    tunnel: w110 -> [w185]
    tunnel: [w185] -> w109
    tunnel: w102 -> [_]
    tunnel: w100 -> [w176]
    tunnel: [w176] -> w99
    tunnel: w61 -> [w177]
    tunnel: [w177] -> w95
    tunnel: [w165] -> w89
    tunnel: w52 -> [w174]
    tunnel: [w174] -> w50
    tunnel: w45 -> [w173]
    tunnel: [w173] -> w44
    tunnel: w10 -> [w165]
    tunnel: [w236] -> w112
    tunnel: w111 -> [w236]
    tunnel: w109 -> [w235]
    tunnel: [w235] -> w108
    tunnel: w99 -> [w233]
    tunnel: w95 -> [w234]
    tunnel: w89 -> [w232]
    tunnel: [w233] -> w88
    tunnel: [w232] -> w87
    tunnel: [w227] -> w81
    tunnel: [w226] -> w80
    tunnel: [w225] -> w79
    tunnel: [w224] -> w78
    tunnel: [w223] -> w51
    tunnel: w50 -> [w223]
    tunnel: w44 -> [w222]
    tunnel: [w222] -> w43
    tunnel: w112 -> [w281]
    tunnel: w108 -> [w277]
    tunnel: [w275] -> w28
    tunnel: [w274] -> w26
    tunnel: w88 -> [w238]
    tunnel: w87 -> [w243]
    tunnel: [w268] -> w24
    tunnel: w81 -> [w265]
    tunnel: w80 -> [w264]
    tunnel: w79 -> [w263]
    tunnel: w78 -> [w262]
    tunnel: [w261] -> w22
    tunnel: w51 -> [w260]
    tunnel: w43 -> [w251]
    tunnel: [w248] -> w20
    tunnel: [w247] -> w18
    tunnel: [w246] -> w17
    tunnel: [w245] -> w16
    tunnel: [w244] -> w15
    tunnel: w28 -> [w599]
    tunnel: [w599] -> w27
    tunnel: w26 -> [w598]
    tunnel: [w598] -> w25
    tunnel: w24 -> [w597]
    tunnel: [w597] -> w23
    tunnel: w22 -> [w596]
    tunnel: [w596] -> w21
    tunnel: w20 -> [w595]
    tunnel: [w595] -> w19
    tunnel: w18 -> [w593]
    tunnel: w17 -> [w592]
    tunnel: w16 -> [w591]
    tunnel: w15 -> [w590]
    tunnel: w27 -> [w681]
    tunnel: [w681] -> w96
    tunnel: w25 -> [w680]
    tunnel: [w680] -> w94
    tunnel: [w679] -> w84
    tunnel: w23 -> [w679]
    tunnel: w21 -> [w618]
    tunnel: [w618] -> w54
    tunnel: w19 -> [w617]
    tunnel: [w617] -> w11
    frame #0 {
      n44 = local read "FileName"() -> (w171:string)
      n45 = local read "dup path"() -> (w168:path)
      n46 = local read "NumChans"() -> (w175:u32)
      n47 = for {
        N: w175 -> [_]
        tunnel: [w215] -> w188 mode=indexing
        tunnel: w171 -> [w214]
        tunnel: w168 -> [w213]
        i -> [w217]
        n48 = Number To Fractional String(number=w217, precision (6)=i16 0) -> (F-format string=w218:string)  [unwired: 2 in]
        n49 = Concatenate Strings(w214, "_achn" ("string"), w218, ".bin" ("string")) -> (w221:string)
        n50 = Build Path(base path=w213, name or relative path=w221) -> (appended path=w215:path)
      }
      n51 = Concatenate Strings(w171, "_EyeCam" ("string"), ".bin" ("string")) -> (w172:string)
      n52 = Concatenate Strings(w171, "_xraw" ("string"), ".bin" ("string")) -> (w184:string)
      n53 = Concatenate Strings(w171, "_ts" ("string"), ".bin" ("string")) -> (w191:string)
      n54 = Build Path(base path=w168, name or relative path=w172) -> (appended path=w167:path)
      n55 = Build Path(base path=w168, name or relative path=w184) -> (appended path=w181:path)
      n56 = Build Path(base path=w168, name or relative path=w191) -> (appended path=w180:path)
      n57 = case shown="False" "SaveData" {
        tunnel: [w197 w208] -> w187
        tunnel: w188 -> [_ w206]
        tunnel: [refnum<file> refnum ("refnum out") w207] -> w179
        tunnel: w181 -> [_ w205]
        tunnel: w180 -> [_ w204]
        tunnel: [refnum<file> refnum ("refnum out") w203] -> w178
        tunnel: w175 -> [w194 _]
        tunnel: w167 -> [_ w202]
        tunnel: [refnum<file> refnum ("refnum out") w199] -> w166
        frame False {
          n58 = for {
            N: w194 -> [_]
            tunnel: [refnum<file> refnum ("refnum out")] -> w197 mode=indexing
          }
        }
        frame True {
          w200 = T14."create" ("operation (0:open)")
          w201 = enum16{"read/write", "read-only", "write-only"}."write-only" ("access (0:read/write)")
          n59 = for {
            tunnel: [w212] -> w208 mode=indexing
            tunnel: w200 -> [w211]
            tunnel: w201 -> [w210]
            tunnel: w206 -> [w209] mode=indexing
            n60 = Open/Create/Replace File(file path (use dialog)=w209, operation (0:open)=w211, access (0:read/write)=w210) -> (refnum out=w212:refnum<file>)  [unwired: 3 in, 2 out]
          }
          n61 = Open/Create/Replace File(file path (use dialog)=w202, operation (0:open)=w200, access (0:read/write)=w201) -> (refnum out=w199:refnum<file>)  [unwired: 3 in, 2 out]
          n62 = Open/Create/Replace File(file path (use dialog)=w205, operation (0:open)=w200, access (0:read/write)=w201) -> (refnum out=w207:refnum<file>)  [unwired: 3 in, 2 out]
          n63 = Open/Create/Replace File(file path (use dialog)=w204, operation (0:open)=w200, access (0:read/write)=w201) -> (refnum out=w203:refnum<file>)  [unwired: 3 in, 2 out]
        }
      }
      n64 = Bundle(w187, "refnum out"=w179, "refnum out"=w178, "refnum out"=w166) -> (w186:T15)  [unwired: 1 in]
    }
    frame #1 {
      n65 = Unbundle(w234) -> ("task out"=w231:refnum<k21>, "error out"=w230:errorcluster, "task out"=w229:refnum<k21>, "error out"=w228:errorcluster)
      n66 = call <vilib>:"DAQmx Start Task.vi"("task/channels in"=w231, "error in"=w230) -> ("task out"=w227:refnum<k21>, "error out"=w226:errorcluster)  [unwired: 12 in]
      n67 = call <vilib>:"DAQmx Start Task.vi"("task/channels in"=w229, "error in"=w228) -> ("task out"=w225:refnum<k21>, "error out"=w224:errorcluster)  [unwired: 12 in]
    }
    frame #2 {
      n68 = disable-structure shown="Disabled" {
        disable-tunnel: w238 -> [w311 _]
        disable-tunnel: [w310 _] -> w273
        disable-tunnel: [w309 _] -> w272
        disable-tunnel: [w308 _] -> w271
        frame Disabled {
          n69 = while {
            tunnel: [w327] -> w309
            tunnel: [w315] -> _
            tunnel: [w312] -> w310
            tunnel: w311 -> [w319]
            tunnel: [w315] -> w308
            stop <- w328 stop-if-true
            w325 = IMAQdx_Buffer_Number_Mode."Next"  # Buffer Number Mode
            n70 = Unbundle(w319) -> ("New Image"=w318:T1, "Session Out"=w317:T3, "error out"=w316:errorcluster)
            n71 = Tick Count (ms)() -> (millisecond timer value=w320:u32)
            n72 = feedback #1() -> (w322:u32)  [unwired: 1 in]
            n73 = feedback-in #1(w320) -> ()
            n74 = Subtract(x=w320, y=w322) -> (x-y=→"Cam1AcqRes[ms]":u32)
            n75 = local read "all stop"() -> (w323:bool)
            n76 = call <vilib>:"IMAQdx Get Image.vi"("Buffer Number Mode (Next)"=w325, "error in"=w316, "Image In"=w318, "Session In"=w317) -> ("error out"=w315:errorcluster, "Buffer Number Out"=w324:u32, "Image Out"=w312:T1, "Session Out"=w327:T3)  [unwired: 1 in, 3 out]
            "Buffer Number" <- w324
            n77 = call "IMAQ Rotate"("Angle (degrees)"=sgl 90.0, "Image Src"=w312) -> ("Image Dst Out"=→"?":T1)  [unwired: 8 in, 1 out]
            n78 = Or(x=w315, y=w323) -> (x .or. y?=w328:bool)
            n79 = call <vilib>:"Calculate Frames per Second.vi"("Buffer Number"=w324) -> ("Processed Frames/s"=→"Frame Rate":dbl)  [unwired: 8 in, 2 out]
          }
        }
        frame Enabled {
        }
      }
      n80 = Tick Count (ms)() -> (millisecond timer value=w266:u32)
      n81 = while {
        shift-right: [w538] -> _
        shift-left: 0.0 -> [w555]
        tunnel: w277 -> [w554]
        tunnel: [w548] -> w276
        tunnel: [w545] -> w274
        tunnel: w266 -> [w527]
        tunnel: w265 -> [w514]
        tunnel: w264 -> [w513]
        tunnel: w263 -> [w512]
        tunnel: w262 -> [w511]
        shift-right: [w488] -> _
        shift-left: _ -> [w494]
        shift-right: [w493] -> _
        shift-left: 0.0 -> [w484]
        i -> [w549]
        stop <- w570 stop-if-true
        n82 = flat-sequence {
          tunnel: [w581] -> w534
          tunnel: [w580] -> w533
          tunnel: [w579] -> w532
          tunnel: [w578] -> w531
          tunnel: [w577] -> w530
          tunnel: [w576] -> w529
          tunnel: w514 -> [w574]
          tunnel: w513 -> [w573]
          tunnel: w512 -> [w572]
          tunnel: w511 -> [w571]
          tunnel: [w584] -> w500
          tunnel: [w585] -> w524
          tunnel: [w586] -> w535
          tunnel: [w587] -> w508
          tunnel: [w588] -> w525
          tunnel: w534 -> [w588]
          tunnel: w533 -> [w587]
          tunnel: w532 -> [w586]
          tunnel: w531 -> [w585]
          tunnel: w530 -> [w584]
          tunnel: [w583] -> w526
          tunnel: [w582] -> w528
          tunnel: w529 -> [w582]
          frame #0 {
            n83 = local read "samples per channel"() -> (w575:i32)
            n84 = call-poly <vilib>:"DAQmx Read.vi"("task/channels in"=w572, "number of samples per channel"=w575, "error in"=w571) -> ("task out"=w576:refnum<k21>, "data"=w580:dbl[], "error out"=w581:errorcluster)  [unwired: 10 in]
            n85 = call-poly <vilib>:"DAQmx Read.vi"("task/channels in"=w574, "number of samples per channel"=w575, "error in"=w573) -> ("task out"=w579:refnum<k21>, "data"=w577:waveform(dbl)[], "error out"=w578:errorcluster)  [unwired: 10 in]
          }
          frame #1 {
            n86 = Tick Count (ms)() -> (millisecond timer value=w583:u32)
          }
        }
        n87 = Index Array(array=w500, index=1) -> (element=w506:waveform(dbl))
        n88 = Index Array(array=w500, index=5) -> (element=w503:waveform(dbl))
        n89 = Unbundle By Name(w506) -> ("Y"=→"LEDDriver":dbl[])
        n90 = Unbundle By Name(w503) -> ("Y"=→"Lick":dbl[])
        n91 = Index Array(array=w508, index=0) -> (element=w510:dbl)
        n92 = Bundle("task out"=w528, "error out"=w525, "task out"=w535, "error out"=w524) -> (w545:T9)  [unwired: 1 in]
        n93 = Index Array(array=w500, index=7) -> (element=w561:waveform(dbl))
        n94 = Index Array(array=w500, index=8) -> (element=w557:waveform(dbl))
        n95 = Index Array(array=w500, index=6) -> (element=w556:waveform(dbl))
        n96 = Index Array(array=w500, index=4) -> (element=w559:waveform(dbl))
        n97 = Index Array(array=w500, index=3) -> (element=w558:waveform(dbl))
        n98 = Index Array(array=w500, index=2) -> (element=w560:waveform(dbl))
        n99 = Index Array(array=w500, index=0) -> (element=w521:waveform(dbl))
        n100 = Subtract(x=w526, y=w527) -> (x-y=w552:u32)
        n101 = Unbundle By Name(w561) -> ("Y"=→"Punish":dbl[])
        n102 = Unbundle By Name(w557) -> ("Y"=→"Reward":dbl[])
        n103 = Unbundle By Name(w556) -> ("Y"=w489:dbl[])
        "Position" <- w489
        n104 = Unbundle By Name(w559) -> ("Y"=w496:dbl[])
        n105 = Unbundle By Name(w558) -> ("Y"=→"Stim ID":dbl[])
        n106 = Unbundle By Name(w560) -> ("Y"=→"Photodiode":dbl[])
        n107 = Unbundle By Name(w521) -> ("Y"=→"FramePulse":dbl[])
        n108 = Greater?(x=w510, y=4000000000.0) -> (0:w540:bool)
        n109 = Index Array(array=w496, index=0) -> (element=→"Speed (tunnel)":dbl)
        n110 = feedback-in #2(w526) -> ()
        n111 = feedback #2() -> (w547:u32)  [unwired: 1 in]
        n112 = Select(t=0.0, s=w540, f=w510) -> (s? t:f=w538:dbl)
        n113 = Subtract(x=w526, y=w547) -> (x-y=→"AcqLoopRes[ms]":u32)
        n114 = Index Array(array=w489, index=0) -> (element=w488:dbl)
        n115 = Divide(x=w552, y=1000) -> (x/y=→"Elapsed time":dbl)
        n116 = Subtract(x=w538, y=w555) -> (x-y=w544:dbl)
        n117 = Subtract(x=w488, y=w494) -> (x-y=w495:dbl)
        n118 = local read "AcqLoopRes[ms]"() -> (w515:u32)
        n119 = Less?(x=w495, y=-4.8) -> (x < y?=w486:bool)
        n120 = Bundle("data"=w500, "data"=w508, "millisecond timer value"=w526, w549) -> (w509:T6)  [unwired: 1 in]
        n121 = Multiply(x=w544, y=0.0157) -> (x*y=w542:dbl)
        n122 = Unbundle By Name(w524) -> ("status"=w568:bool)
        n123 = Unbundle By Name(w525) -> ("status"=w569:bool)
        n124 = Merge Errors(w525, w524) -> (→"error out":errorcluster)
        n125 = Select(t=1.0, s=w486, f=0.0) -> (s? t:f=w485:dbl)
        n126 = Enqueue Element(queue=w554, element=w509) -> (queue out=w548:refnum<queue>)  [unwired: 2 in, 2 out]
        n127 = Add(x=w485, y=w484) -> (x+y=w493:dbl)
        "Number of trials" <- w493
        n128 = local read "all stop"() -> (w553:bool)
        n129 = Compound Arithmetic op=OR(w569, w568, w553) -> (w570:bool)
        n130 = Divide(x=w515, y=1000) -> (x/y=w499:dbl)
        n131 = Divide(x=w542, y=w499) -> (x/y=→"Speed":dbl)
        "AIAcqLoop" <- w549
      }
      n132 = disable-structure shown="Enabled" {
        disable-tunnel: w243 -> [w285 _]
        disable-tunnel: [w284 _] -> w242
        disable-tunnel: [w283 _] -> w241
        disable-tunnel: [w282 _] -> w240
        frame Enabled {
          n133 = node-c288() -> (w287:T11)  [unwired: 4 in]
          n134 = timed-loop {
            tunnel: w285 -> [w295]
            tunnel: [w290] -> w283
            tunnel: [w291] -> w282
            tunnel: [w289] -> w284
            timing: w287 -> [_]
            timing-out: [_] -> w286
            i -> [w288]
            stop <- w303 stop-if-true
            w301 = IMAQdx_Buffer_Number_Mode."Next"  # Buffer Number Mode
            n135 = node-c288() -> ()  [unwired: 1 in, 1 out]
            n136 = Tick Count (ms)() -> (millisecond timer value=w296:u32)
            n137 = feedback #3() -> (w297:u32)  [unwired: 1 in]
            n138 = feedback-in #3(w296) -> ()
            n139 = Unbundle(w295) -> ("New Image"=w294:T1, "Session Out"=w293:T3, "error out"=w292:errorcluster)
            n140 = Subtract(x=w296, y=w297) -> (x-y=→"Cam2AcqRes[ms]":u32)
            n141 = local read "all stop"() -> (w299:bool)
            n142 = call <vilib>:"IMAQdx Get Image.vi"("Buffer Number Mode (Next)"=w301, "error in"=w292, "Image In"=w294, "Session In"=w293) -> ("error out"=w290:errorcluster, "Buffer Number Out"=w300:u32, "Image Out"=w291:T1, "Session Out"=w289:T3)  [unwired: 1 in, 3 out]
            "?" <- w291
            "Buffer Number  2" <- w300
            n143 = Or(x=w290, y=w299) -> (x .or. y?=w303:bool)
            n144 = call <vilib>:"Calculate Frames per Second.vi"("Buffer Number"=w300) -> ("Processed Frames/s"=→"Frame Rate 2":dbl)  [unwired: 8 in, 2 out]
            n145 = node-c288() -> ()  [unwired: 1 in, 1 out]
            "Numeric 2" <- w288
          }
          n146 = node-c288(w286) -> ()  [unwired: 1 out]
        }
        frame Disabled {
        }
      }
      n147 = Unbundle(w260) -> ("Session Out"=w256:T3, "New Image"=w255:T1, "New Image"=w252:T1, "error out"=w259:errorcluster)
      n148 = node-c288() -> (w254:T11)  [unwired: 4 in]
      n149 = timed-loop "Eyecamera" {
        tunnel: w259 -> [w391]
        tunnel: [w390] -> w258
        tunnel: [w388] -> w257
        tunnel: w251 -> [w384]
        tunnel: w256 -> [w383]
        tunnel: w255 -> [w382]
        timing: w254 -> [_]
        timing-out: [_] -> w253
        tunnel: w252 -> [w378]
        tunnel: [w380] -> w249
        tunnel: [w378] -> w239
        i -> [w386]
        stop <- w389 stop-if-true
        w367 = 1 ("X Step Size")
        w373 = 5 items=["Red", "Green", "Blue", "Hue", "Saturation", "Luminance", "Value", "Intensity"] ("Color Plane")
        n150 = node-c288() -> ()  [unwired: 1 in, 1 out]
        n151 = call <vilib>:"IMAQdx Grab.vi"("error in"=w391, "Image In"=w382, "Session In"=w383) -> ("error out"=w392:errorcluster, "Buffer Number Out"=w385:u32, "Image Out"=w393:T1, "Session Out"=w381:T3)  [unwired: 1 in, 4 out]
        n152 = call <vilib>:"Calculate Frames per Second.vi"("Buffer Number"=w385) -> ("Acquired Frames/s"=→"Acquired Frames CAM0":dbl)  [unwired: 8 in, 2 out]
        n153 = flat-sequence {
          tunnel: [w407] -> w387
          tunnel: w392 -> [w406]
          tunnel: [w406] -> w388
          tunnel: [w405] -> w379
          tunnel: w393 -> [w405]
          tunnel: w381 -> [w404]
          tunnel: [w404] -> w390
          frame #0 {
            n154 = Tick Count (ms)() -> (millisecond timer value=w407:u32)
          }
        }
        n155 = Unbundle By Name(w388) -> ("status"=w376:bool)
        n156 = local read "all stop"() -> (w375:bool)
        n157 = call "IMAQ ExtractSingleColorPlane"("Color Plane"=w373, "Image Dst"=w378, "Image Src"=w379) -> ("Image Dst Out"=w365:T1)  [unwired: 7 in, 1 out]
        n158 = Or(x=w376, y=w375) -> (x .or. y?=w389:bool)
        n159 = call "IMAQ Extract 2"("Y Step Size"=w367, "Optional Rectangle"="Optional Rectangle", "X Step Size"=w367, "Image Src"=w365) -> ("Image Dst Out"=w369:T1)  [unwired: 6 in, 1 out]
        n160 = property class="IMAQImage" props=["ImageSize", "ImageName", "ImageType"](reference=w369) -> (reference out=w368:T1, "ImageSize"=→"Image Size":cluster{"x":i32, "y":i32}, "ImageType"=→"Image Type":i32)  [unwired: 1 in, 2 out]
        "Image CAM0- front view 2" <- w368
        n161 = call "IMAQ ImageToArray"("Image"=w368) -> ("Image Pixels (U8)"=w374:u8[][])  [unwired: 3 in, 4 out]
        n162 = local read "SaveData"() -> (w366:bool)
        n163 = case shown="True" w366 {
          tunnel: w374 -> [_ w398]
          tunnel: w387 -> [_ w400]
          tunnel: w386 -> [_ w401]
          tunnel: w385 -> [_ w399]
          tunnel: w384 -> [w394 w396]
          tunnel: [w394 w395] -> w380
          frame False {
          }
          frame True {
            n164 = Bundle(w401, "millisecond timer value"=w400, "Buffer Number Out"=w399, "Image Pixels (U8)"=w398) -> (w397:T5)  [unwired: 1 in]
            n165 = Enqueue Element(queue=w396, element=w397) -> (queue out=w395:refnum<queue>)  [unwired: 2 in, 2 out]
          }
        }
        n166 = node-c288() -> ()  [unwired: 1 in, 1 out]
        "Image CAM0- front view 3" <- w379
        "Numeric" <- w386
      }
      n167 = Bundle("Image Out"=w240, "Session Out"=w242, "error out"=w241) -> (w269:T17)  [unwired: 1 in]
      n168 = Unbundle(w281) -> (w280:refnum<file>[], "refnum out"=w279:refnum<file>, "refnum out"=w278:refnum<file>, "refnum out"=w250:refnum<file>)
      n169 = while "Write Timestamps  Loop" {
        tunnel: [w432] -> w247
        tunnel: [w427] -> w246
        tunnel: w280 -> [w425]
        tunnel: w279 -> [w424]
        tunnel: w278 -> [w423]
        tunnel: [w422] -> w245
        tunnel: w277 -> [w421]
        i -> [w417]
        stop <- w426 stop-if-true
        n170 = Dequeue Element(queue=w421) -> (element=w416:T6, error out=w426:errorcluster)  [unwired: 2 in, 2 out]
        n171 = Tick Count (ms)() -> (millisecond timer value=w420:u32)
        n172 = Unbundle(w416) -> ("data"=w430:waveform(dbl)[], "data"=w415:dbl[], "millisecond timer value"=w413:u32, w411:i32)
        n173 = feedback #4() -> (w419:u32)  [unwired: 1 in]
        n174 = feedback-in #4(w420) -> ()
        n175 = To Double Precision Float(number=w415) -> (double precision float=w414:dbl[])
        n176 = To Double Precision Float(number=w413) -> (double precision float=w412:dbl)
        n177 = To Double Precision Float(number=w411) -> (double precision float=w410:dbl)
        n178 = Subtract(x=w420, y=w419) -> (x-y=→"SaveLoopRes[ms]":u32)
        n179 = Index Array(array=w430, index=0) -> (element=w429:waveform(dbl))
        n180 = Unbundle By Name(w429) -> ("t0"=w428:timestamp)
        n181 = case shown="No Error" w426 {
          tunnel: [w436 w471] -> w432
          tunnel: w412 -> [w444 _]
          tunnel: w430 -> [w443 _]
          tunnel: w428 -> [w442 _]
          tunnel: w414 -> [w441 _]
          tunnel: [w440 w470] -> w427
          tunnel: w410 -> [w439 _]
          tunnel: w425 -> [w438 w471]
          tunnel: w424 -> [w437 w470]
          tunnel: w423 -> [w435 w469]
          tunnel: [w434 w469] -> w422
          frame No Error {
            n182 = local read "SaveData"() -> (w433:bool)
            n183 = case shown="True" w433 {
              tunnel: w444 -> [_ w454]
              tunnel: w443 -> [_ w460]
              tunnel: w442 -> [_ w459]
              tunnel: [w447 w458] -> w436
              tunnel: w441 -> [_ w456]
              tunnel: [w446 w455] -> w440
              tunnel: w439 -> [_ w453]
              tunnel: w438 -> [w447 w452]
              tunnel: w437 -> [w446 w451]
              tunnel: [w445 w450] -> w434
              tunnel: w435 -> [w445 w449]
              frame False {
              }
              frame True {
                w457 = T2."big-endian, network order" ("byte order (0:big-endian, network order)")
                w448 = FALSE ("append to file? (new file:F)")
                n184 = for {
                  tunnel: w460 -> [w468] mode=indexing
                  tunnel: w448 -> [w465]
                  tunnel: [w464] -> w458 mode=indexing
                  tunnel: w452 -> [w463] mode=indexing
                  n185 = Unbundle By Name(w468) -> ("Y"=w467:dbl[])
                  n186 = To Single Precision Float(number=w467) -> (single precision float=w466:sgl[])
                  n187 = Write to Binary File(file (use dialog)=w463, data=w466, 5:w465) -> (refnum out=w464:refnum<file>)  [unwired: 3 in, 2 out]
                }
                n188 = Write to Binary File(file (use dialog)=w449, data=w459, 5:w448, 9:w457) -> (refnum out=w462:refnum<file>)  [unwired: 2 in, 2 out]
                n189 = Write to Binary File(file (use dialog)=w462, data=w454, 5:w448, 9:w457) -> (refnum out=w461:refnum<file>)  [unwired: 2 in, 2 out]
                n190 = Write to Binary File(file (use dialog)=w451, data=w456, 5:w448, 9:w457) -> (refnum out=w455:refnum<file>)  [unwired: 2 in, 2 out]
                n191 = Write to Binary File(file (use dialog)=w461, data=w453, 5:w448, 9:w457) -> (refnum out=w450:refnum<file>)  [unwired: 2 in, 2 out]
                "byte order (0:big-endian, network order)" <- w457
              }
            }
          }
          frame Error {
          }
        }
        "AISaveLoop" <- w417
      }
      n192 = while "Write Timestamps  Loop" {
        tunnel: w251 -> [w334]
        tunnel: w250 -> [w331]
        tunnel: [w330] -> w244
        i -> [w340]
        stop <- w344 stop-if-true
        n193 = Dequeue Element(queue=w334) -> (element=w339:T5, error out=w344:errorcluster)  [unwired: 2 in, 2 out]
        n194 = Tick Count (ms)() -> (millisecond timer value=w343:u32)
        n195 = Unbundle(w339) -> (w333:i32, "millisecond timer value"=w338:u32, "Buffer Number Out"=w336:u32, "Image Pixels (U8)"=w332:u8[][])
        n196 = feedback #5() -> (w342:u32)  [unwired: 1 in]
        n197 = feedback-in #5(w343) -> ()
        n198 = To Unsigned Long Integer(number=w338) -> (unsigned 32bit integer=w337:u32)
        n199 = To Unsigned Long Integer(number=w336) -> (unsigned 32bit integer=w335:u32)
        n200 = To Unsigned Long Integer(number=w333) -> (unsigned 32bit integer=w329:u32)
        n201 = Subtract(x=w343, y=w342) -> (x-y=→"SaveLoopRes[ms] 2":u32)
        n202 = case shown="No Error" w344 {
          tunnel: w335 -> [w351 _]
          tunnel: w337 -> [w350 _]
          tunnel: w332 -> [w349 _]
          tunnel: w331 -> [w348 w364]
          tunnel: [w347 w364] -> w330
          tunnel: w329 -> [w346 _]
          frame No Error {
            n203 = local read "SaveData"() -> (w345:bool)
            n204 = case shown="True" w345 {
              tunnel: w351 -> [_ w355]
              tunnel: w350 -> [_ w356]
              tunnel: w349 -> [_ w354]
              tunnel: w348 -> [w352 w361]
              tunnel: [w352 w358] -> w347
              tunnel: w346 -> [_ w357]
              frame False {
              }
              frame True {
                w353 = T2."big-endian, network order" ("byte order (0:big-endian, network order) 2")
                w362 = FALSE ("append to file? (new file:F)")
                n205 = Write to Binary File(file (use dialog)=w361, data=w357, 5:w362, 9:w353) -> (refnum out=w363:refnum<file>)  [unwired: 2 in, 2 out]
                n206 = Write to Binary File(file (use dialog)=w363, data=w356, 5:w362, 9:w353) -> (refnum out=w360:refnum<file>)  [unwired: 2 in, 2 out]
                n207 = Write to Binary File(file (use dialog)=w360, data=w355, 5:w362, 9:w353) -> (refnum out=w359:refnum<file>)  [unwired: 2 in, 2 out]
                n208 = Write to Binary File(file (use dialog)=w359, data=w354, 5:w362, 9:w353) -> (refnum out=w358:refnum<file>)  [unwired: 2 in, 2 out]
              }
            }
          }
          frame Error {
          }
        }
        "AISaveLoop 2" <- w340
      }
      n209 = Bundle("Session Out"=w258, "error out"=w257, "New Image"=w239) -> (w261:T18)  [unwired: 1 in]
      n210 = node-c288(w253) -> ()  [unwired: 1 out]
      n211 = Bundle("Image Out"=w273, "Session Out"=w272, "error out"=w271) -> (w270:T17)  [unwired: 1 in]
      n212 = while {
        tunnel: [w480] -> w275
        tunnel: w276 -> [w479]
        tunnel: w249 -> [w476]
        tunnel: [w472] -> w248
        stop <- w481 stop-if-true
        n213 = Get Queue Status(queue=w479) -> (queue out=w478:refnum<queue>, # elements in queue=w477:i32)  [unwired: 2 in, 6 out]
        "# elements in queue" <- w477
        n214 = Get Queue Status(queue=w476) -> (queue out=w473:refnum<queue>, # elements in queue=w475:i32)  [unwired: 2 in, 6 out]
        "# elements in queue 2" <- w475
        n215 = local read "all stop"() -> (w482:bool)
        n216 = Equal To 0?(x=w475) -> (x = 0?=w474:bool)
        n217 = Equal To 0?(x=w477) -> (x = 0?=w483:bool)
        n218 = Compound Arithmetic op=AND(w482, w483, w474) -> (w481:bool)
        n219 = Release Queue(queue=w478) -> (error out=w480:errorcluster)  [unwired: 2 in, 2 out]
        n220 = Release Queue(queue=w473) -> (error out=w472:errorcluster)  [unwired: 2 in, 2 out]
      }
      n221 = Bundle(w270, w269) -> (w268:T19)  [unwired: 1 in]
    }
    frame #3 {
      n222 = local read "SaveData"() -> (w589:bool)
      n223 = case shown="True" w589 {
        tunnel: w590 -> [_ w600]
        frame False {
        }
        frame True {
          n224 = Close File(refnum=w600) -> ()  [unwired: 1 in, 2 out]
        }
      }
      n225 = local read "SaveData"() -> (w594:bool)
      n226 = case shown="True" w594 {
        tunnel: w593 -> [_ w603]
        tunnel: w592 -> [_ w602]
        tunnel: w591 -> [_ w601]
        frame False {
        }
        frame True {
          n227 = for {
            tunnel: w603 -> [w604] mode=indexing
            n228 = Close File(refnum=w604) -> ()  [unwired: 1 in, 2 out]
          }
          n229 = Close File(refnum=w602) -> ()  [unwired: 1 in, 2 out]
          n230 = Close File(refnum=w601) -> ()  [unwired: 1 in, 2 out]
        }
      }
    }
    frame #4 {
      w605 = "EyeCam" ("key")
      w622 = "_ts" ("section")
      w638 = "_xraw" ("section")
      w648 = "_achn" ("section")
      w657 = "Binnary" ("section")
      w662 = "AI" ("section")
      n231 = local read "Image Size"() -> (w612:cluster{"x":i32, "y":i32})
      n232 = Unbundle By Name(w612) -> ("x"=w608:i32, "y"=w607:i32)
      n233 = local read "FileName"() -> (w678:string)
      n234 = local read "dup path"() -> (w675:path)
      n235 = Current VI's Path() -> (path=w624:path)
      n236 = Path To String(path=w624) -> (string=w623:string)
      n237 = Concatenate Strings(w678, "_log.ini" ("string")) -> (w676:string)
      n238 = Build Path(base path=w675, name or relative path=w676) -> (appended path=w674:path)
      n239 = local read "samples per channel"() -> (w619:i32)
      n240 = local read "AIAcqLoop"() -> (w659:i32)
      n241 = call <vilib>:"Open Config Data.vi"("configuration file path"=w674) -> ("refnum"=w673:T20)  [unwired: 8 in, 2 out]
      n242 = local read "byte order (0:big-endian, network order)"() -> (w658:T2)
      n243 = local read "AISaveLoop"() -> (w660:i32)
      n244 = local read "NumChans"() -> (w621:u32)
      n245 = call-poly <vilib>:"Write Key.vi"("section"=w662, "value"=w621, "key"="NCh" ("section"), "refnum"=w673) -> ("refnum out"=w669:T20)  [unwired: 5 in, 2 out]
      n246 = local read "rate"() -> (w620:dbl)
      n247 = call-poly <vilib>:"Write Key.vi"("section"=w662, "value"=w620, "key"="Rate" ("section"), "refnum"=w669) -> ("refnum out"=w668:T20)  [unwired: 5 in, 2 out]
      n248 = call-poly <vilib>:"Write Key.vi"("section"=w662, "value"=w619, "key"="NSmp" ("section"), "refnum"=w668) -> ("refnum out"=w661:T20)  [unwired: 5 in, 2 out]
      n249 = call-poly <vilib>:"Write Key.vi"("section"=w657, "value"=w660, "key"="AISave" ("section"), "refnum"=w661) -> ("refnum out"=w666:T20)  [unwired: 5 in, 2 out]
      n250 = call-poly <vilib>:"Write Key.vi"("section"=w657, "value"=w659, "key"="AIAcq" ("section"), "refnum"=w666) -> ("refnum out"=w667:T20)  [unwired: 5 in, 2 out]
      n251 = call-poly <vilib>:"Write Key.vi"("section"=w657, "value"=w658, "key"="Order" ("section"), "refnum"=w667) -> ("refnum out"=w652:T20)  [unwired: 5 in, 2 out]
      n252 = call-poly <vilib>:"Write Key.vi"("section"=w648, "value"=1, "key"="NCh", "refnum"=w652) -> ("refnum out"=w651:T20)  [unwired: 5 in, 2 out]
      n253 = call-poly <vilib>:"Write Key.vi"("section"=w648, "value"="SGL" ("key"), "key"="Type", "refnum"=w651) -> ("refnum out"=w650:T20)  [unwired: 5 in, 2 out]
      n254 = call-poly <vilib>:"Write Key.vi"("section"=w648, "value"=32, "key"="Size [Bit]", "refnum"=w650) -> ("refnum out"=w639:T20)  [unwired: 5 in, 2 out]
      n255 = call-poly <vilib>:"Write Key.vi"("section"=w638, "value"=1, "key"="NCh", "refnum"=w639) -> ("refnum out"=w637:T20)  [unwired: 5 in, 2 out]
      n256 = call-poly <vilib>:"Write Key.vi"("section"=w638, "value"="DBL" ("key"), "key"="Type", "refnum"=w637) -> ("refnum out"=w644:T20)  [unwired: 5 in, 2 out]
      n257 = call-poly <vilib>:"Write Key.vi"("section"=w638, "value"=64, "key"="Size [Bit]", "refnum"=w644) -> ("refnum out"=w628:T20)  [unwired: 5 in, 2 out]
      n258 = call-poly <vilib>:"Write Key.vi"("section"=w622, "value"=4, "key"="NCh", "refnum"=w628) -> ("refnum out"=w636:T20)  [unwired: 5 in, 2 out]
      n259 = call-poly <vilib>:"Write Key.vi"("section"=w622, "value"="DBL" ("key"), "key"="Type", "refnum"=w636) -> ("refnum out"=w631:T20)  [unwired: 5 in, 2 out]
      n260 = call-poly <vilib>:"Write Key.vi"("section"=w622, "value"=64, "key"="Size [Bit]", "refnum"=w631) -> ("refnum out"=w615:T20)  [unwired: 5 in, 2 out]
      n261 = call-poly <vilib>:"Write Key.vi"("section"=w605, "value"=w608, "key"="sizeX", "refnum"=w615) -> ("refnum out"=w610:T20)  [unwired: 5 in, 2 out]
      n262 = call-poly <vilib>:"Write Key.vi"("section"=w605, "value"=w607, "key"="sizeY", "refnum"=w610) -> ("refnum out"=w609:T20)  [unwired: 5 in, 2 out]
      n263 = local read "Image Type"() -> (w606:i32)
      "Image Type 2" <- w606
      n264 = call-poly <vilib>:"Write Key.vi"("section"=w605, "value"=w606, "key"="Type", "refnum"=w609) -> ("refnum out"=w613:T20)  [unwired: 5 in, 2 out]
      n265 = call-poly <vilib>:"Write Key.vi"("section"="General" ("key"), "value"=w623, "key"="VI", "refnum"=w613) -> ("refnum out"=w625:T20)  [unwired: 5 in, 2 out]
      n266 = call <vilib>:"Close Config Data.vi"("refnum"=w625) -> ()  [unwired: 9 in, 2 out]
    }
  }
  n267 = Unbundle(w84) -> (w83:T17, w82:T17)
  n268 = disable-structure shown="Disabled" {
    disable-tunnel: [w692 _] -> w97
    disable-tunnel: w82 -> [w691 _]
    disable-tunnel: [w690 _] -> w8
    frame Disabled {
      w690 = TRUE
      n269 = Unbundle(w691) -> ("Image Out"=w684:T1, "Session Out"=w683:T3, "error out"=w682:errorcluster)
      n270 = call <vilib>:"IMAQdx Stop Acquisition.vi"("error in"=w682, "Session In"=w683) -> ("error out"=w688:errorcluster, "Session Out"=w687:T3)  [unwired: 8 out]
      n271 = call <vilib>:"IMAQdx Unconfigure Acquisition.vi"("error in"=w688, "Session In"=w687) -> ("error out"=w685:errorcluster, "Session Out"=w686:T3)  [unwired: 8 out]
      n272 = call <vilib>:"IMAQdx Close Camera.vi"("error in"=w685, "Session In"=w686) -> ("error out"=w689:errorcluster)  [unwired: 9 out]
      n273 = call "IMAQ Dispose"("All Images? (No)"=w690, "Image"=w684, "error in (no error)"=w689) -> ("error out"=w692:errorcluster)  [unwired: 3 in]
    }
    frame Enabled {
    }
  }
  n274 = disable-structure shown="Disabled" {
    disable-tunnel: [w703 _] -> w98
    disable-tunnel: w83 -> [w702 _]
    disable-tunnel: w8 -> [w693 _]
    frame Disabled {
      n275 = Unbundle(w702) -> ("Image Out"=w696:T1, "Session Out"=w695:T3, "error out"=w694:errorcluster)
      n276 = call <vilib>:"IMAQdx Stop Acquisition.vi"("error in"=w694, "Session In"=w695) -> ("error out"=w698:errorcluster, "Session Out"=w699:T3)  [unwired: 8 out]
      n277 = call <vilib>:"IMAQdx Unconfigure Acquisition.vi"("error in"=w698, "Session In"=w699) -> ("error out"=w701:errorcluster, "Session Out"=w700:T3)  [unwired: 8 out]
      n278 = call <vilib>:"IMAQdx Close Camera.vi"("error in"=w701, "Session In"=w700) -> ("error out"=w697:errorcluster)  [unwired: 9 out]
      n279 = call "IMAQ Dispose"("All Images? (No)"=w693, "Image"=w696, "error in (no error)"=w697) -> ("error out"=w703:errorcluster)  [unwired: 3 in]
    }
    frame Enabled {
    }
  }
  n280 = Unbundle(w54) -> ("Session Out"=w48:T3, "error out"=w39:errorcluster, "New Image"=w9:T1)
  n281 = Unbundle(w94) -> ("task out"=w93:refnum<k21>, "error out"=w92:errorcluster, "task out"=w91:refnum<k21>, "error out"=w90:errorcluster)
  n282 = flat-sequence {
    tunnel: w48 -> [w705]
    tunnel: [w705] -> w49
    tunnel: w49 -> [w711]
    tunnel: [w708] -> w12
    tunnel: w39 -> [w707]
    tunnel: w9 -> [w706]
    frame #0 {
      n283 = Wait (ms)(milliseconds to wait=u32 200) -> ()  [unwired: 1 out]
    }
    frame #1 {
      n284 = call <vilib>:"IMAQdx Close Camera.vi"("error in"=w707, "Session In"=w711) -> ("error out"=w709:errorcluster)  [unwired: 9 out]
      n285 = call "IMAQ Dispose"("All Images? (No)"=TRUE, "Image"=w706, "error in (no error)"=w709) -> ("error out"=w708:errorcluster)  [unwired: 3 in]
    }
  }
  n286 = call <vilib>:"DAQmx Stop Task.vi"("task/channels in"=w93, "error in"=w92) -> ("task out"=w104:refnum<k21>, "error out"=w103:errorcluster)  [unwired: 12 in]
  n287 = call <vilib>:"DAQmx Stop Task.vi"("task/channels in"=w91, "error in"=w90) -> ("task out"=w107:refnum<k21>, "error out"=w106:errorcluster)  [unwired: 12 in]
  n288 = call <vilib>:"DAQmx Clear Task.vi"("task in"=w104, "error in"=w103) -> ("error out"=w86:errorcluster)  [unwired: 13 in]
  n289 = call <vilib>:"DAQmx Clear Task.vi"("task in"=w107, "error in"=w106) -> ("error out"=w85:errorcluster)  [unwired: 13 in]
  n290 = Merge Errors(w86, w85, w96, w98, w97, w12, w11) -> (w105:errorcluster)
  "CamerasOK? TaskEnd OK?" <- w105
  n291 = call <vilib>:"General Error Handler.vi"("error in (no error)"=w105) -> ()  [unwired: 10 in, 5 out]
